vi "Initialization VI.vi"(8 "error in (no error)":errorcluster, 10 "Custom XML":string, 11 "Device Item Ref in":T1 format="%.0x") -> (0 "error out":errorcluster, 3 "Device Item Ref out":T1 format="%.0x")   [LabVIEW 2014, in "SLSC configuration System Explorer.lvlib"]
uses:
  SLSC configuration System Explorer.lvlib
  <vilib>/NI Veristand/Custom Device API/Custom Device Item Ref.ctl
  Shared/Type Defs/RIO Device Address.ctl
  Shared/Constants.vi
  <vilib>/NI Veristand/Custom Device API/Set Item Property (U32).vi
  <vilib>/NI Veristand/Custom Device API/Set Item Property (String).vi
  <vilib>/NI Veristand/Custom Device API/Set Item Property (U16).vi
  <vilib>/NI Veristand/Custom Device API/Custom Device API.lvlib
  Shared/SLSC configuration Shared.lvlib
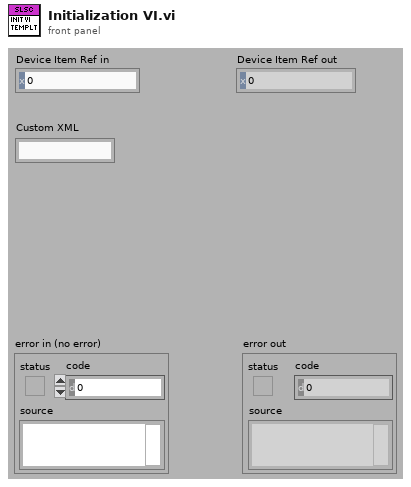
[diagram p1: front panel]
types:
  T1 = typedef "Custom Device API.lvlib/Custom Device Item Ref.ctl" = u64
  T2 = typedef "SLSC configuration System Explorer.lvlib/RIO Device Address.ctl" = string
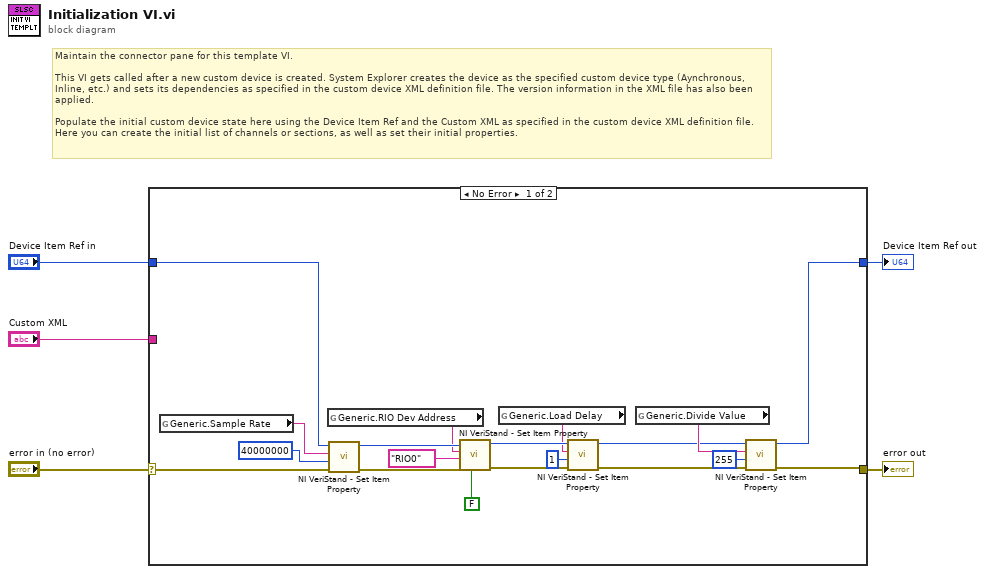
[diagram p0: block diagram]
diagram:
  # "Maintain the connector pane for this template VI.\n\nThis VI gets called after a new custom device is created. System Explorer creates the device as the specified custom device type (Aynchronous, Inline, etc.) and sets its dependencies as specified in the custom device XML definition file. The version information in the XML file has also been applied.\n\nPopulate the initial custom device state here using the Device Item Ref and the Custom XML as specified in the custom device XML definition file. Here you can create the initial list of channels or sections, as well as set their initial properties."
  n1 = case shown="No Error" "error in (no error)" {
    selector: "error in (no error)" -> [w21 w26]
    tunnel: [w8 w26] -> w5
    tunnel: [w7 w25] -> w3
    tunnel: "Device Item Ref in" -> [w22 w25]
    tunnel: "Custom XML" -> [_ _]
    frame No Error {
      n2 = global read "Constants.vi" "Generic.Sample Rate"() -> (w24:string)
      n3 = global read "Constants.vi" "Generic.RIO Dev Address"() -> (w17:string)
      n4 = call-poly <vilib>:"NI VeriStand - Set Item Property.vi"("error in (no error)"=w21, "Value"=u32 40000000, "Property Name"=w24, "Item Ref in"=w22) -> ("error out"=w19:errorcluster, "Item Ref out"=w18:T1)  [unwired: 5 in, 1 out]
      n5 = call-poly <vilib>:"NI VeriStand - Set Item Property.vi"("Binary String (T)"=FALSE, "error in (no error)"=w19, "Value"=T2 "RIO0" ("RIO Device Address"), "Property Name"=w17, "Item Ref in"=w18) -> ("error out"=w15:errorcluster, "Item Ref out"=w14:T1)  [unwired: 4 in, 1 out]
      n6 = global read "Constants.vi" "Generic.Load Delay"() -> (w13:string)
      n7 = call-poly <vilib>:"NI VeriStand - Set Item Property.vi"("error in (no error)"=w15, "Value"=u16 1, "Property Name"=w13, "Item Ref in"=w14) -> ("error out"=w10:errorcluster, "Item Ref out"=w9:T1)  [unwired: 5 in, 1 out]
      n8 = global read "Constants.vi" "Generic.Divide Value"() -> (w11:string)
      n9 = call-poly <vilib>:"NI VeriStand - Set Item Property.vi"("error in (no error)"=w10, "Value"=u16 255, "Property Name"=w11, "Item Ref in"=w9) -> ("error out"=w8:errorcluster, "Item Ref out"=w7:T1)  [unwired: 5 in, 1 out]
    }
    frame Error {
    }
  }
  "error out" <- w5
  "Device Item Ref out" <- w3
